vi "CD Write Engine.vi"(0 "Input Channel Data []":T5[](array[typedef]) {"Labels Settings"."Label Timestamp Channel Data Reference" format="%.0x"; "Labels Settings"."Label Disable/Trigger Channel Reference" format="%.0x"; "Labels Settings"."Word"."Param Setting"."Item Refs" format="%.0x"; "Labels Settings"."Word"."Param Setting"."Num Bits" min=1 max=32; "Labels Settings"."Word"."Param Setting"."Start Bit" min=8 max=31; "Labels Settings"."Label" format="%.0o"}, 5 "Data (in)":dbl[](array[numeric]), 11 "Error (in)":errorcluster, 12 "Raw Values":T1, 13 "Map":T4[](array[typedef]) {"Channel Data Reference" format="%.0x"}) -> (6 "Data (out)":dbl[](array[numeric]), 15 "Error (out)":errorcluster)   [LabVIEW 2016, in "Ballard Arinc-429 Engine.lvlib"]
uses:
  Ballard Arinc-429 Engine.lvlib
  Shared/Controls and Global/Label.ctl
  Shared/Ballard Arinc-429 Shared.lvlib
  Shared/Controls and Global/transferPeriod.ctl
  Shared/Controls and Global/Start Bit.ctl
  Shared/Controls and Global/Number of Bits.ctl
  Shared/Controls and Global/RT Param Setting.ctl
  Shared/Controls and Global/TransferType.ctl
  Shared/Controls and Global/RT HW Channel.ctl
  RT Controls/RT Tx Association.ctl
  RT Controls/RT Tx Default Raw Value_Association.ctl
  RT Controls/RT Tx Default Raw Value.ctl
  Shared/Controls and Global/RT Word Settings.ctl
  Shared/Controls and Global/RT Label Settings.ctl
  <vilib>/NI Veristand/Custom Device API/Data Reference.ctl
  <vilib>/NI VeriStand/Custom Device API/Custom Device API.lvlib
  <vilib>/NI Veristand/Custom Device API/Block Data Reference.ctl
  <vilib>/NI Veristand/Custom Device API/Custom Device Item Ref.ctl
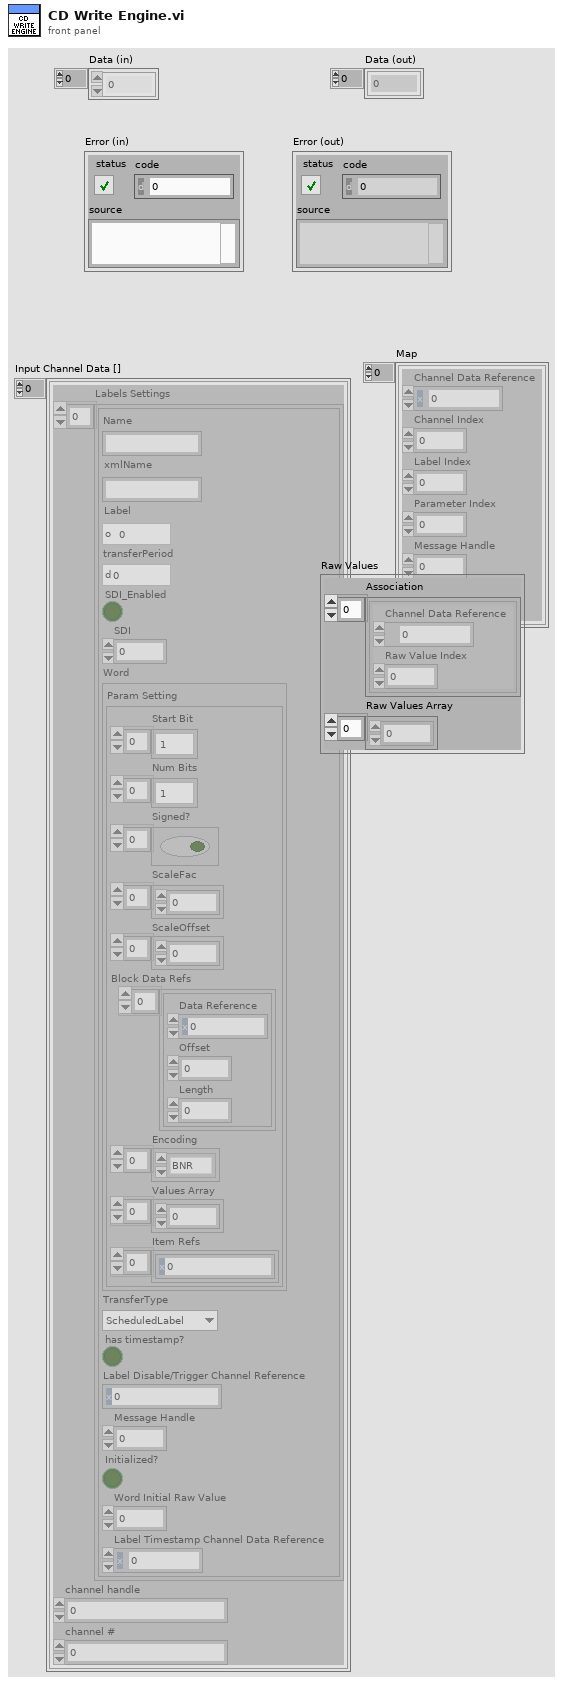
[diagram p1: front panel]
types:
  T1 = typedef "Ballard Arinc-429 Engine.lvlib/RT Tx Default Raw Value.ctl" = cluster{"Association":T2[], "Raw Values Array":u32[]}
  T2 = typedef "Ballard Arinc-429 Engine.lvlib/RT Tx Default Raw Value_Association.ctl" = cluster{"Channel Data Reference":T3, "Raw Value Index":i32}
  T3 = typedef "Custom Device API.lvlib/Data Reference.ctl" = i32
  T4 = typedef "Ballard Arinc-429 Engine.lvlib/RT Tx Association.ctl" = cluster{"Channel Data Reference":T3, "Channel Index":i32, "Label Index":i32, "Parameter Index":i32, "Message Handle":u64, "Type":enum16{"Parameter Channel", "Disable/Trigger Channel"}}
  T5 = typedef "Ballard Arinc-429 Shared.lvlib/RT HW Channel.ctl" = cluster{"Labels Settings":T6[], "channel handle":u64, "channel #":u16}
  T6 = typedef "Ballard Arinc-429 Shared.lvlib/RT Label Settings.ctl" = cluster{"Name":string, "xmlName":string, "Label":T7, "transferPeriod":T8, "SDI_Enabled":bool, "SDI":u8, "Word":T9, "TransferType":T15, "has timestamp?":bool, "Label Disable/Trigger Channel Reference":T14, "Message Handle":u64, "Initialized?":bool, "Word Initial Raw Value":u32, "Label Timestamp Channel Data Reference":T3}
  T7 = typedef "Ballard Arinc-429 Shared.lvlib/Label.ctl" = u8
  T8 = typedef "Ballard Arinc-429 Shared.lvlib/transferPeriod.ctl" = u32
  T9 = typedef "Ballard Arinc-429 Shared.lvlib/RT Word Settings.ctl" = cluster{"Param Setting":T10}
  T10 = typedef "Ballard Arinc-429 Shared.lvlib/RT Param Setting.ctl" = cluster{"Start Bit":T11[], "Num Bits":T12[], "Signed?":bool[], "ScaleFac":dbl[], "ScaleOffset":dbl[], "Block Data Refs":T13[], "Encoding":enum16{"BNR", "BCD", "Discrete"}[], "Values Array":dbl[], "Item Refs":T14[]}
  T11 = typedef "Ballard Arinc-429 Shared.lvlib/Start Bit.ctl" = i32
  T12 = typedef "Ballard Arinc-429 Shared.lvlib/Number of Bits.ctl" = i32
  T13 = typedef "Custom Device API.lvlib/Block Data Reference.ctl" = cluster{"Data Reference":T3, "Offset":u64, "Length":u64}
  T14 = typedef "Custom Device API.lvlib/Custom Device Item Ref.ctl" = u64
  T15 = typedef "Ballard Arinc-429 Shared.lvlib/TransferType.ctl" = enum16{"ScheduledLabel", "Acyclic", "Block", "Strobe"}
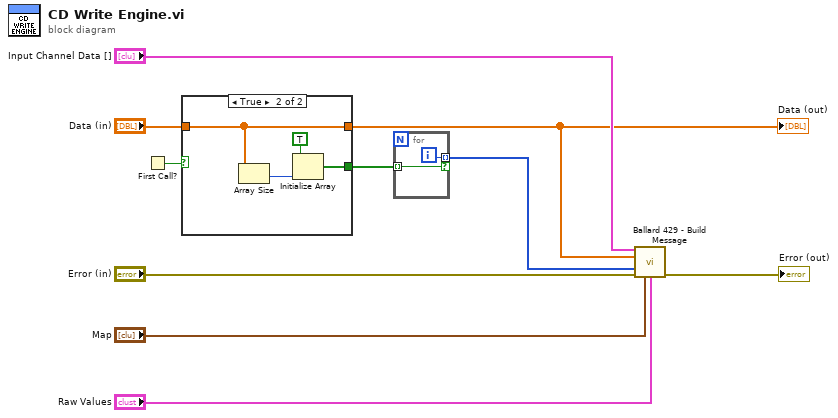
[diagram p0: block diagram]
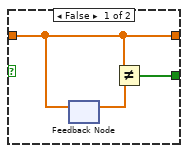
[diagram p2: hidden frame]
diagram:
  n1 = First Call?() -> (First Call?: T/F=w3:bool)
  n2 = case shown="True" w3 {
    tunnel: "Data (in)" -> [w11 w17]
    tunnel: [w12 w14] -> w5
    tunnel: [w11 w17] -> w4
    frame False {
      n3 = feedback #1() -> (w13:dbl[])  [unwired: 1 in]
      n4 = feedback-in #1(w11) -> ()
      n5 = Not Equal?(x=w11, y=w13) -> (x != y?=w12:bool[])
    }
    frame True {
      n6 = Array Size(array=w17) -> (size(s)=w16:i32)
      n7 = Initialize Array(TRUE, w16) -> (w14:bool[])
    }
  }
  "Data (out)" <- w4
  n8 = for {
    tunnel: w5 -> [w19] mode=indexing
    tunnel: [w18] -> w6 mode=indexing if=w19
    i -> [w18]
  }
  n9 = call "Ballard 429 - Build Message.vi"("Channel Data []"="Input Channel Data []", "Doubles []"=w4, "Updated FIFO Index []"=w6, "Error (in)"="Error (in)", "Map"="Map", "Raw Values"="Raw Values") -> ("Error (out)"=→"Error (out)":errorcluster)  [unwired: 9 in]
